vi "ROI entry-Select whole plane.vi"() -> (0 "error IO":errorcluster)   [LabVIEW 2020]
uses:
  Typedefs/ROI management FG states.ctl
  Typedefs/ROI ID Enum.ctl
  ROI Entry screen/Typedefs/Redraw ROI.ctl
  <resource>/objmgr/IMAQImage.rc
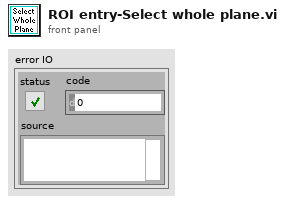
[diagram p1: front panel]
types:
  T1 = typedef "IMAQ Image.ctl" = refnum<image>
  T2 = typedef "ROI management FG states.ctl" = enum16{"Read", "Write", "Write-from dataset", "Clear Last", "Clear All", "Delete ROI", "Update ROIs time", "Reload last ROI set", "Modify ROI Parameters", "Offset all ROI", "Offset visible ROI", "Modify Dwell Time", "Modify Laser Power"}
  T3 = typedef "Redraw ROI.ctl" = enum16{"Redraw All", "Redraw Deselected", "Draw Last", "Redraw Selected"}
  T4 = typedef "ROI ID Enum.ctl" = enum16{"Point", "MiniScan", "Comp. MiniScan", "Rectangle", "Comp. volume", "Arb. plane point", "None"}
  T5 = typedef "ROI parameters data type.ctl" = cluster{"ROI index":dbl, "ROI ID":dbl, "ROI Time (ns)":dbl, "Pixels in ROI":dbl, "X start":dbl, "Y start":dbl, "Z start":dbl, "X stop":dbl, "Y stop":dbl, "Z stop":dbl, "Angle (deg)":dbl, "Composite ID":dbl, "Number of lines":dbl, "Frame Size":dbl, "Zoom":dbl, "Laser Power (%)":dbl, "ROI group ID":dbl, "Resolution":dbl, "Dwell Time per pixel":dbl, "Pixels per miniscan":dbl, "Original FOV (um)":dbl, "Apparent Frame Size":dbl, "Z Plane Idx":i32[], "Z Plane codes":i32[]}
  T6 = typedef "ROI Z-stack settings info.ctl" = cluster{"Zoom":dbl, "POI Dwell time":dbl, "Rel. Res":dbl, "Laser Power %":dbl, "Frame Size":dbl, "FOV":dbl}
  T7 = typedef "ROI spec.ctl" = cluster{"ROI Enum":T4, "Coordinates":i32[], "Zoom":dbl, "POI Dwell time":dbl, "Rel. Resolution":dbl, "Laser Power":dbl, "Frame Size":dbl, "FOV":dbl, "Z start":dbl, "Z stop":dbl, "Z planeIdx(s)":i32[], "Z planecodes(s)":u8[]}
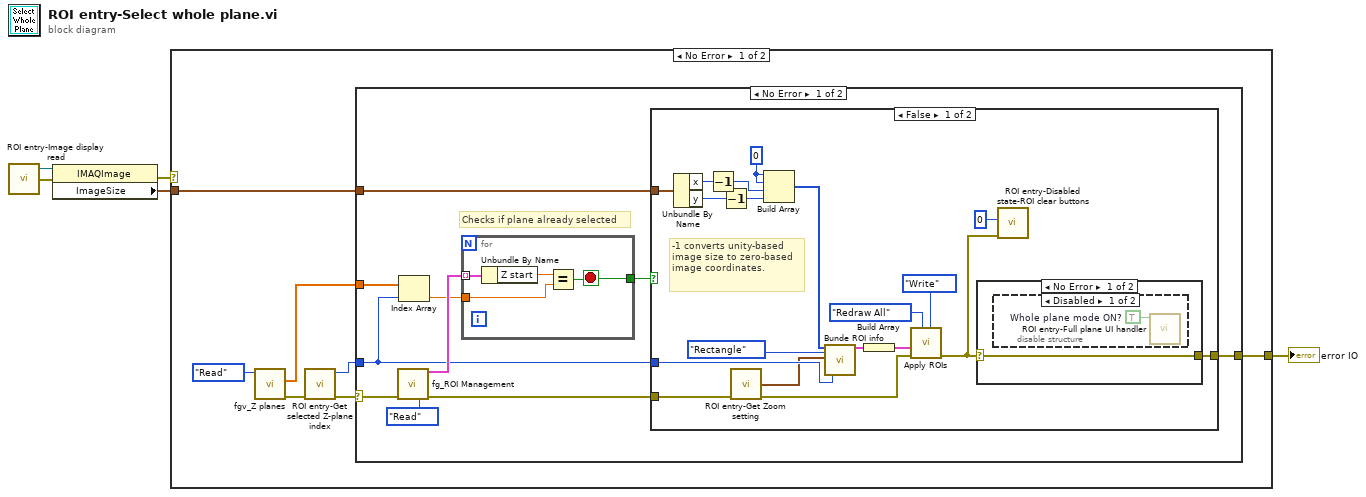
[diagram p0: block diagram]
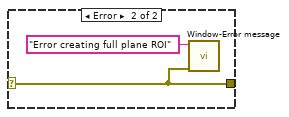
[diagram p3: hidden frame]
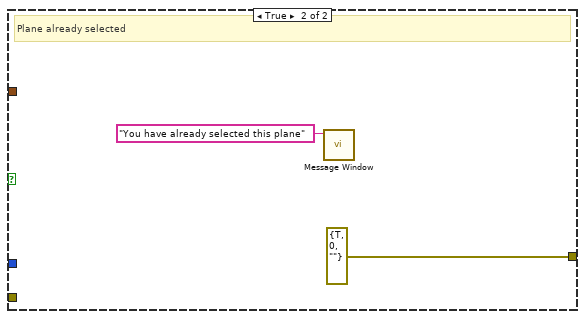
[diagram p4: hidden frame]
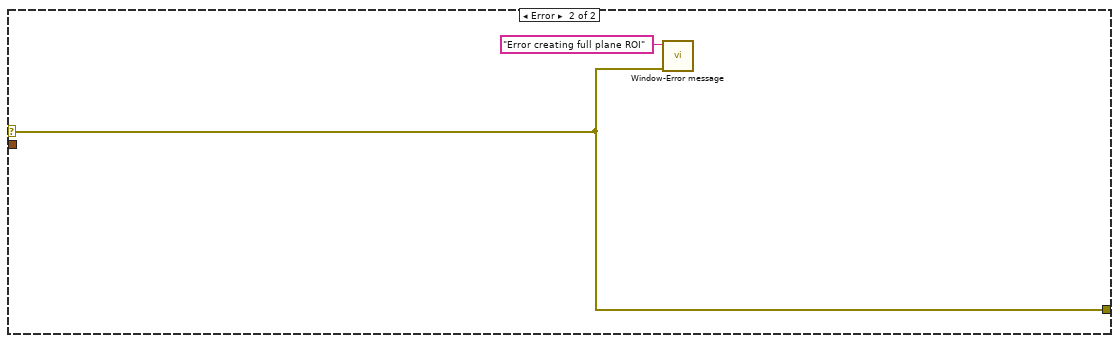
[diagram p6: hidden frame]
diagram:
  n1 = call "ROI entry-Image display read.vi"() -> ("error out"=w1:errorcluster, "CurrentImage"=w2:T1)  [unwired: 4 in]
  n2 = property class="IMAQImage"(reference=w2, error in=w1) -> (error out=w4:errorcluster, "ImageSize"=w5:cluster{"x":i32, "y":i32})  [unwired: 1 out]
  n3 = case shown="No Error" w4 {
    selector: w4 -> [_ w53]
    tunnel: w5 -> [w12 _]
    tunnel: [w11 w53] -> w3
    frame No Error {
      n4 = call "fgv_Z planes.vi"("Function"=enum16{"Intialize", "Write", "Read", "Clear"}."Read") -> ("error out"=w7:errorcluster, "AOL Z Planes"=w9:dbl[])  [unwired: 8 in, 1 out]
      n5 = call "ROI entry-Get selected Z-plane index.vi"("error in (no error)"=w7) -> ("error out"=w6:errorcluster, "Z-plane selector (index)"=w8:i32)  [unwired: 9 in]
      n6 = case shown="No Error" w6 {
        selector: w6 -> [w14 w52]
        tunnel: w12 -> [w18 _]
        tunnel: [w17 w52] -> w11
        tunnel: w9 -> [w16 _]
        tunnel: w8 -> [w15 _]
        frame No Error {
          # "Checks if plane already selected"
          n7 = call "fg_ROI Management.vi"("Function"=ROI_management_FG_states."Read", "error in (no error)"=w14) -> ("ROI Setup"=w21:T5[], "error out"=w13:errorcluster)  [unwired: 7 in, 5 out]
          n8 = Index Array(array=w16, index=w15) -> (element=w20:dbl)
          n9 = for {
            tunnel: w21 -> [w51] mode=indexing
            tunnel: w20 -> [w49]
            tunnel: [w48] -> w19
            stop <- w48 stop-if-true
            n10 = Unbundle By Name(w51) -> ("Z start"=w50:dbl)
            n11 = Equal?(x=w50, y=w49) -> (x = y?=w48:bool)
          }
          n12 = case shown="False" w19 {
            tunnel: w18 -> [w36 _]
            tunnel: w15 -> [w26 _]
            tunnel: [w35 errorcluster {"status"=TRUE, "code"=0, "source"=""} ("error IO")] -> w17
            tunnel: w13 -> [w33 _]
            frame False {
              w40 = 0
              # "-1 converts unity-based image size to zero-based image coordinates."
              n13 = Unbundle By Name(w36) -> ("x"=w38:i32, "y"=w37:i32)
              n14 = Decrement(x=w38) -> (x-1=w29:i32)
              n15 = Decrement(x=w37) -> (x-1=w28:i32)
              n16 = call "ROI entry-Get Zoom setting.vi"("error in (no error)"=w33) -> ("AOLZ Settings"=w25:T6, "error out"=w34:errorcluster)  [unwired: 6 in, 7 out]
              n17 = Build Array(w40, w40, w29, w28) -> (w30:i32[])
              n18 = call "Bunde ROI info.vi"("ROI Coordinates"=w30, "ROI Enum"=ROI_ID_Enum."Rectangle", "Z stack Settings"=w25, "ZplaneIndex"=w26) -> ("ROI Info"=w41:T7)  [unwired: 15 in]
              n19 = Build Array(w41) -> (w39:T7[])
              n20 = call "Apply ROIs.vi"("Function"=ROI_management_FG_states."Write", "Mode (Redraw All)"=Redraw_ROI."Redraw All", "error in (no error)"=w34, "ROIs Info []"=w39) -> ("error out"=w23:errorcluster)  [unwired: 5 in, 2 out]
              n21 = case shown="No Error" w23 {
                selector: w23 -> [w42 w44]
                tunnel: [w42 w44] -> w35
                frame No Error {
                  n22 = disable-structure shown="Disabled" {
                    frame Disabled {
                      w43 = TRUE  # Whole plane mode ON?
                      n23 = call "ROI entry-Full plane UI handler.vi"("Whole plane mode ON"=w43) -> ()  [unwired: 10 in, 1 out]
                    }
                    frame Enabled {
                    }
                  }
                }
                frame Error {
                  n24 = call "Window-Error message.vi"("error in (no error)"=w44, "Message"="Error creating full plane ROI") -> ()  [unwired: 9 in, 1 out]
                }
              }
              n25 = call "ROI entry-Disabled state-ROI clear buttons.vi"("error in (no error)"=w23, "State"=0) -> ()  [unwired: 9 in, 1 out]
            }
            frame True {
              # "Plane already selected"
              n26 = call "Message Window.vi"("Message string"="You have already selected this plane") -> ()  [unwired: 10 in, 1 out]
            }
          }
        }
        frame Error {
        }
      }
    }
    frame Error {
      n27 = call "Window-Error message.vi"("error in (no error)"=w53, "Message"="Error creating full plane ROI") -> ()  [unwired: 9 in, 1 out]
    }
  }
  "error IO" <- w3
